vi "Is Created Attribute.vi"(9 "Alias":string, 10 "Map of Created Attributes":T1) -> (1 "Created Attributes":refnum<class "Attributes.lvclass">, 2 "Error":errorcluster)   [LabVIEW 2020, in "jettl.lvlib" / "Actor.lvlib"]
uses:
  Actor.lvlib
  Created Attributes Map.ctl
  Attributes/Attributes/Attributes.lvclass
  Error/Error.lvlib
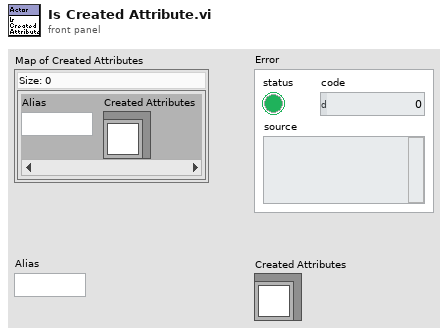
[diagram p1: front panel]
types:
  T1 = typedef "jettl.lvlib/Actor.lvlib/Created Attributes Map.ctl" = map{string, refnum<class "Attributes.lvclass">}
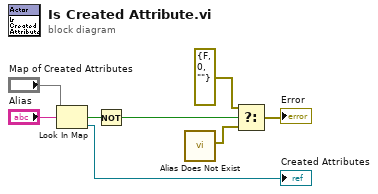
[diagram p0: block diagram]
diagram:
  n1 = Look In Map(map="Map of Created Attributes", key="Alias") -> (key not found?=w2:bool, value=→"Created Attributes":refnum<class "Attributes.lvclass">)  [unwired: 1 in]
  n2 = Not(x=w2) -> (.not. x?=w1:bool)
  n3 = call "Alias Does Not Exist.vi"() -> ("Error"=w6:errorcluster)  [unwired: 11 in]
  n4 = Select(t=errorcluster {"status"=FALSE, "code"=0, "source"=""}, s=w1, f=w6) -> (s? t:f=→"Error":errorcluster)
